vi "GetResult.vi"(3 "measurements":cluster{"id":u32, "passed":bool}[](array[cluster])) -> (0 "passed":bool, 1 "id":u32)   [LabVIEW 2019]
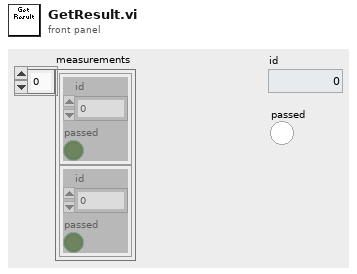
[diagram p1: front panel]
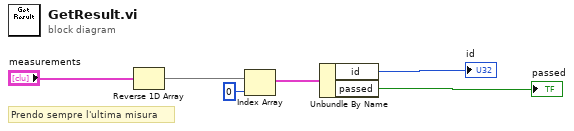
[diagram p0: block diagram]
diagram:
  # "Prendo sempre l'ultima misura"
  n1 = Reverse 1D Array(array="measurements") -> (reversed array=w5:cluster{"id":u32, "passed":bool}[])
  n2 = Index Array(array=w5, index=0) -> (element=w3:cluster{"id":u32, "passed":bool})
  n3 = Unbundle By Name(w3) -> ("id"=→"id":u32, "passed"=→"passed":bool)
